vi "对应优化算法.vi"(8 "散斑图像作用结果优化":dbl[](array[numeric]), 9 "筛选门限":dbl, 10 "光源散斑簇":T2, 11 "模块选择簇":T1) -> (2 "作用结果筛选数":dbl, 3 "散斑图像作用结果（处理）":dbl[][](array[numeric]))   [LabVIEW 2018]
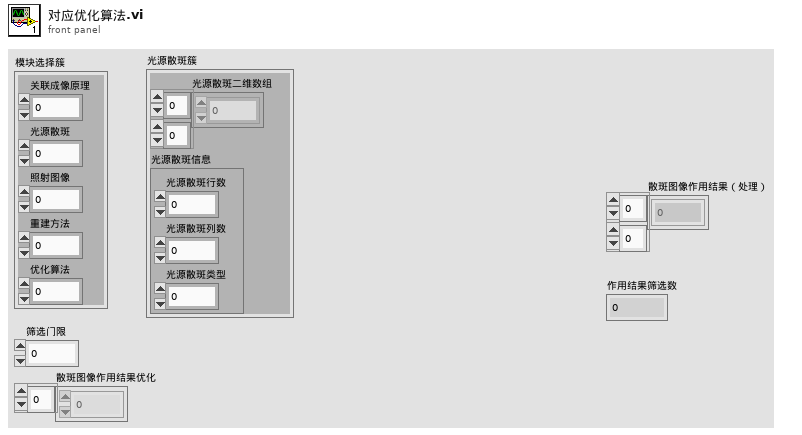
[diagram p1: front panel]
types:
  T1 = cluster{"关联成像原理":i32, "光源散斑":i32, "照射图像":i32, "重建方法":i32, "优化算法":i32}
  T2 = cluster{"光源散斑二维数组":dbl[][], "光源散斑信息":cluster{"光源散斑行数":dbl, "光源散斑列数":dbl, "光源散斑类型":dbl}}
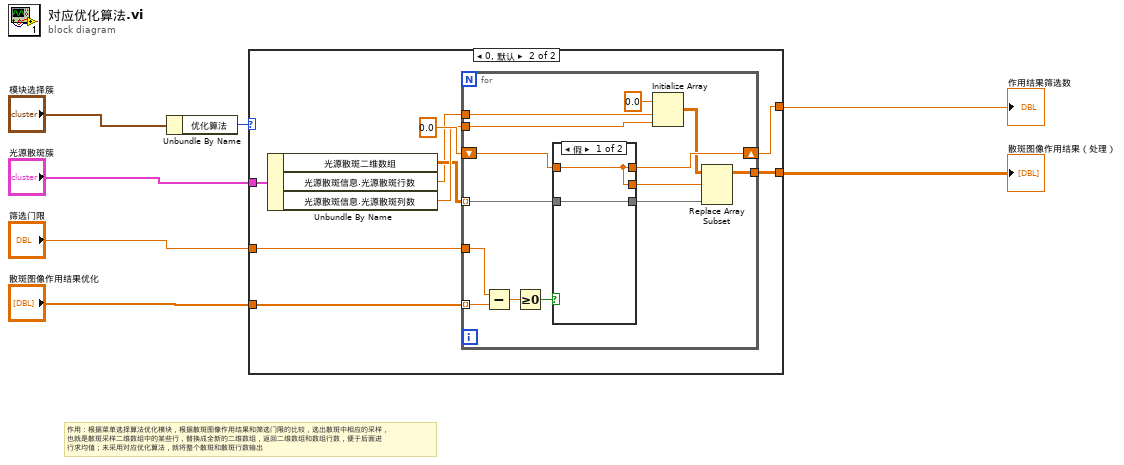
[diagram p0: block diagram]
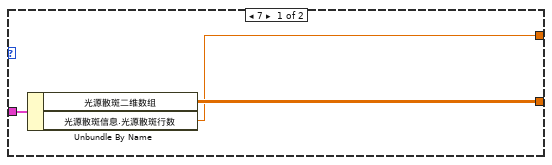
[diagram p2: hidden frame]
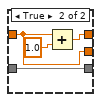
[diagram p3: hidden frame]
diagram:
  # "作用：根据菜单选择算法优化模块，根据散斑图像作用结果和筛选门限的比较，选出散斑中相应的采样，\n也就是散斑采样二维数组中的某些行，替换成全新的二维数组，返回二维数组和数组行数，便于后面进\n行求均值；未采用对应优化算法，就将整个散斑和散斑行数输出"
  n1 = Unbundle By Name("模块选择簇") -> ("优化算法"=w6:i32)
  n2 = case shown="0, 默认" w6 {
    tunnel: "光源散斑簇" -> [w10 w19]
    tunnel: [w9 w13] -> w4
    tunnel: [w8 w11] -> w3
    tunnel: "筛选门限" -> [_ w18]
    tunnel: "散斑图像作用结果优化" -> [_ w17]
    frame 7 {
      n3 = Unbundle By Name(w10) -> ("光源散斑二维数组"=w9:dbl[][], "光源散斑信息.光源散斑行数"=w8:dbl)
    }
    frame 0, Default {
      n4 = Unbundle By Name(w19) -> ("光源散斑二维数组"=w14:dbl[][], "光源散斑信息.光源散斑行数"=w12:dbl, "光源散斑信息.光源散斑列数"=w15:dbl)
      n5 = for {
        tunnel: w18 -> [w33]
        tunnel: w17 -> [w32] mode=indexing
        shift-right: [w28] -> w11
        shift-left: 0.0 -> [w29]
        tunnel: w15 -> [w24]
        tunnel: w14 -> [w27] mode=indexing
        tunnel: [w20] -> w13
        tunnel: w12 -> [w25]
        n6 = Subtract(x=w33, y=w32) -> (x-y=w31:dbl)
        n7 = Greater Or Equal To 0?(x=w31) -> (x >= 0?=w30:bool)
        n8 = case shown="假" w30 {
          tunnel: [w35 w39] -> w21
          tunnel: w29 -> [w35 w39]
          tunnel: [w35 w37] -> w28
          tunnel: [w34 w36] -> w22
          tunnel: w27 -> [w34 w36]
          frame False {
          }
          frame True {
            n9 = Add(x=w39, y=1.0) -> (x+y=w37:dbl)
          }
        }
        n10 = Initialize Array(0.0, w25, w24) -> (w23:dbl[][])
        n11 = Replace Array Subset(array=w23, new element=w22, index (row)=w21) -> (w20:dbl[][])  [unwired: 1 in]
      }
    }
  }
  "散斑图像作用结果（处理）" <- w4
  "作用结果筛选数" <- w3
